vi "Actor Core.vi"(8 "error in":errorcluster, 11 "CS++TestMotor in":refnum<class "CS++TestMotor.lvclass">) -> (0 "error out":errorcluster, 3 "Actor out":refnum<class "Actor.lvclass">)   [LabVIEW 2015, in "CS++TestMotor.lvlib" / "CS++TestMotor.lvclass"]
doc: "(<B>Filename</B>: Actor Framework.lvlib:Actor.lvclass:Actor Core.vi)\n\nReceives messages to the actor, reacts to them, and initiates any error handling that may shut the actor down.\n\nDescendant classes may override this VI to append parallel tasks for the actor to complete while it handles messages. Overrides use the Call Parent Method node."
uses:
  CS++TestMotor.lvclass
  <vilib>/ActorFramework/Actor/Actor.lvclass
  CSPP_Core/Actors/CS++BaseActor/CS++BaseActor.lvclass/CS++BaseActor.ctl
  CS++TestMotor.lvclass/CS++TestMotor.ctl
  CSPP_Core/Classes/CS++BaseClasses/Factory/CS++Factory.lvclass
  CSPP_Core/Actors/CS++BaseActor/CS++BaseActor.lvclass
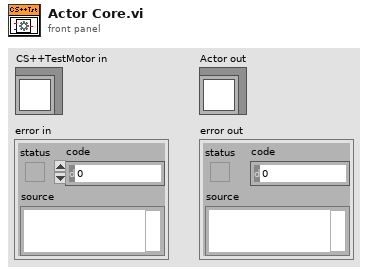
[diagram p1: front panel]
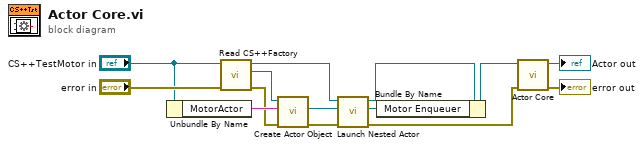
[diagram p0: block diagram]
diagram:
  n1 = Unbundle By Name("CS++TestMotor in") -> ("MotorActor"=w8:string)
  n2 = call "Read CS++Factory.vi"("error in (no error)"="error in", "CS++BaseActor in"="CS++TestMotor in") -> ("error out"=w7:errorcluster, "CS++Factory"=w6:refnum<class "CS++Factory.lvclass">, "CS++BaseActor out"=w12:refnum<class "CS++TestMotor.lvclass">)  [unwired: 7 in]
  n3 = call "Create Actor Object.vi"("error in (no error)"=w7, "Object Name"=w8, "CS++Factory in"=w6) -> ("error out"=w9:errorcluster, "CS++BaseActor"=w10:refnum<class "CS++BaseActor.lvclass">)  [unwired: 5 in, 2 out]
  n4 = call <vilib>:"Launch Nested Actor.vi"("error in (no error)"=w9, "Nested Actor"=w10, "Caller Actor in"=w12) -> ("error out"=w3:errorcluster, "Nested Actor's Enqueuer"=w11:refnum<class "Message Enqueuer.lvclass">, "Caller Actor out"=w13:refnum<class "CS++TestMotor.lvclass">)  [unwired: 6 in]
  n5 = Bundle By Name(cluster=w13, "Motor Enqueuer"=w11) -> (w4:refnum<class "CS++TestMotor.lvclass">)
  n6 = call-parent "Actor Core.vi"("error in"=w3, "CS++BaseActor in"=w4) -> ("error out"=→"error out":errorcluster, "Actor out"=→"Actor out":refnum<class "Actor.lvclass">)  [unwired: 8 in]
